vi "Get Active Devices from Device List.vi"(8 "Error In":errorcluster, 11 "Device List State":T1) -> (0 "Error Out":errorcluster, 2 "Active Devices":refnum<class "Device.lvclass">[](array[class]), 3 "Device List State out":T1)   [LabVIEW 2015]
uses:
  Device List State.ctl
  Device/Device.lvclass
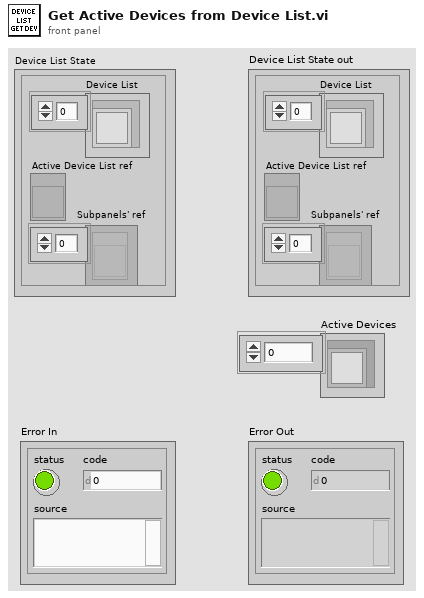
[diagram p1: front panel]
types:
  T1 = typedef "Device List State.ctl" = cluster{"Device List":refnum<class "Device.lvclass">[], "Active Device List ref":refnum<vi>, "Subpanels' ref":refnum<vi>[]}
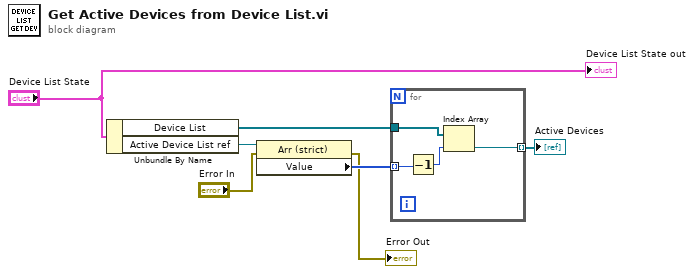
[diagram p0: block diagram]
diagram:
  n1 = Unbundle By Name("Device List State") -> ("Device List"=w5:refnum<class "Device.lvclass">[], "Active Device List ref"=w6:refnum<vi>)
  n2 = property class="Arr (strict)"(reference=w6, error in="Error In") -> (error out=→"Error Out":errorcluster, "Value"=w4:u16[])  [unwired: 1 out]
  n3 = for {
    tunnel: w5 -> [w11]
    tunnel: w4 -> [w10] mode=indexing
    tunnel: [w8] -> w3 mode=indexing
    n4 = Decrement(x=w10) -> (x-1=w9:u16)
    n5 = Index Array(array=w11, index=w9) -> (element=w8:refnum<class "Device.lvclass">)
  }
  "Active Devices" <- w3
  "Device List State out" <- "Device List State"
